vi "VCI Close Device.vi"(10 "DevIndex":u32, 11 "DevType":u32) -> (3 "function return":u32)   [LabVIEW 2010, in "ControlCAN.lvlib"]
doc: "unsigned int WINAPI VCI_CloseDevice(unsigned int DevType,unsigned int DevIndex);"
uses:
  ControlCAN.lvlib
  ControlCAN/Ginkgo_Driver.dll
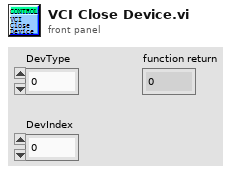
[diagram p1: front panel]
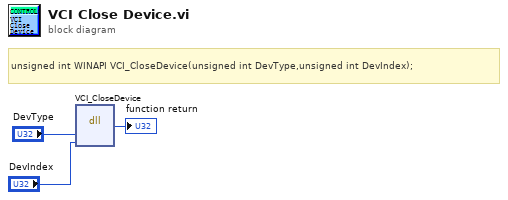
[diagram p0: block diagram]
diagram:
  # "unsigned int WINAPI VCI_CloseDevice(unsigned int DevType,unsigned int DevIndex);"
  n1 = dll-call lib="E:/Project/vt_ginkgo/truck/Ginkgo Driver/vs2010/Ginkgo_USB-I2C&SPI&CAN_API_v2.0.3.3/lib/labview_32bit/ControlCAN/Ginkgo_Driver.*" fn="VCI_CloseDevice"("DevType"="DevType", "DevIndex"="DevIndex") -> (→"function return":u32)  [unwired: 5 in, 2 out]
